vi "ZMQ Rep Test.vi"() -> ()   [LabVIEW 2019, in "RemoteControl.ZMQ.lvclass"]
uses:
  RemoteControl.ZMQ.lvclass
panel:
  out "Command":string
  out "ID":string
  out "Data":variant
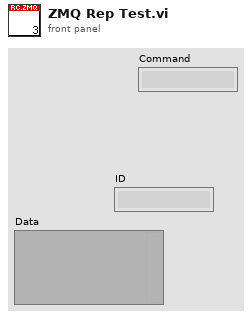
[diagram p1: front panel]
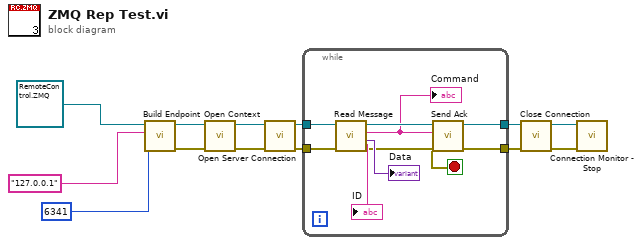
[diagram p0: block diagram]
diagram:
  n1 = call "Build Endpoint.vi"("Port"=u16 6341, "Address"="127.0.0.1", "RemoteControl.ZMQ in"=refnum<class "RemoteControl.ZMQ.lvclass"> refnum ("RemoteControl.ZMQ.lvclass")) -> ("error out"=w8:errorcluster, "RemoteControl.ZMQ out"=w9:refnum<class "RemoteControl.ZMQ.lvclass">)  [unwired: 7 in]
  n2 = call-dynamic "Open Context.vi"("error in (no error)"=w8, "RemoteControl.ZMQ in"=w9) -> ("error out"=w12:errorcluster, "RemoteControl.ZMQ out"=w13:refnum<class "RemoteControl.ZMQ.lvclass">)  [unwired: 8 in]
  n3 = call-dynamic "Open Server Connection.vi"("error in (no error)"=w12, "RemoteControl.ZMQ in"=w13) -> ("error out"=w10:errorcluster, "RemoteControl.ZMQ out"=w11:refnum<class "RemoteControl.ZMQ.lvclass">)  [unwired: 8 in]
  n4 = while {
    tunnel: w11 -> [w22]
    tunnel: [w17] -> w5
    tunnel: w10 -> [w21]
    tunnel: [w14] -> w4
    stop <- w14 stop-if-true
    n5 = call-dynamic "Read Message.vi"("error in (no error)"=w21, "RemoteControl.ZMQ in"=w22) -> ("error out"=w16:errorcluster, "Data"=→"Data":variant, "Command"=w15:string, "RemoteControl.ZMQ out"=w18:refnum<class "RemoteControl.ZMQ.lvclass">, "ID"=→"ID":string)  [unwired: 5 in]
    "Command" <- w15
    n6 = call "Send Ack.vi"("error in (no error)"=w16, "Command Received"=w15, "RemoteControl.ZMQ in"=w18) -> ("error out"=w14:errorcluster, "RemoteControl.ZMQ out"=w17:refnum<class "RemoteControl.ZMQ.lvclass">)  [unwired: 7 in]
  }
  n7 = call-dynamic "Close Connection.vi"("error in (no error)"=w4, "RemoteControl.ZMQ in"=w5) -> ("error out"=w3:errorcluster, "RemoteControl.ZMQ out"=w2:refnum<class "RemoteControl.ZMQ.lvclass">)  [unwired: 8 in]
  n8 = call-dynamic "Connection Monitor - Stop.vi"("error in (no error)"=w3, "RemoteControl.ZMQ in"=w2) -> ()  [unwired: 8 in, 2 out]
